vi "Module_p_control_sing_v3.vi"() -> ()   [LabVIEW 2014]
uses:
  <vilib>/rvi/FXPMathLib/FxpSinAndCos/XNode/nifxpmath_SinAndCos.xnode
  <vilib>/eio/EIONode/EIONode.xnode
  <vilib>/rvi/FXPMathLib/FxpMul/XNode/nifxpmath_Multiplier.xnode
  <vilib>/rvi/FXPMathLib/FxpSinAndCos/simVIs/DllFxpSinAndCosTemp_sub.vi
  <vilib>/rvi/FXPMathLib/FxpSinAndCos/subVIs/nifxpmath_SinAndCos_SimConfig.ctl
  <vilib>/rvi/eio/common/nirviEmuTemplateMethod_errors.vi
  <vilib>/rvi/FXPMathLib/sim/FxpSim.dll
  <vilib>/rvi/DataTransferAndStorage/Container/XNode/niFpgaContainer.xnode
  <vilib>/rvi/FXPMathLib/FxpSub/XNode/nifxpmath_Sub.xnode
  <vilib>/rvi/FXPMathLib/FxpAdd/XNode/nifxpmath_Add.xnode
  <vilib>/rvi/Analysis/measure/butterworth/XNode/niFpgaButterworthFilter.xnode
  <vilib>/rvi/FXPMathLib/FxpAtan2/XNode/nifxpmath_Atan2.xnode
  <vilib>/rvi/FXPMathLib/FxpAtan2/simVIs/DllFxpAtan2Temp_sub.vi
  <vilib>/rvi/FXPMathLib/FxpAtan2/subVIs/nifxpmath_Atan2_SimConfig.ctl
  <vilib>/rvi/interface/RandomDataEmulation/nirviRandomDataFpgaMultiElementTemplate.vi
panel:
  in  "fb_limit":fxp<+,16,11>
  in  "Db_d_M_avg_Tc (uSec)":u32 caption="M_avg_Tc (uSec)"
  in  "Method case 2":i32
  out "Omega_b(rad/s)":fxp<+/-,32,18>
  out "Omega_b(M_avg)":fxp<+/-,32,18>
  out "Omega_b(M)":fxp<+/-,32,18>
  in  "Count(s)":u32
  out "Boolean":bool
  out "Db_temp":fxp<+/-,22,7>
  in  "Sin ini":bool
  out "xb_dd":fxp<+/-,25,15>
  in  "scaled coefficients_xb_dd":i32[](array[numeric])=[1067016412, 3362706]
  out "Db_dd":fxp<+/-,25,15>
  in  "scaled coefficients_Db_dd":i32[](array[numeric])=[1067016412, 3362706]
  out "Dab_edd":fxp<+/-,34,12>
  out "Dab_ed":fxp<+/-,33,10>
  out "fbr":fxp<+/-,20,10>
  in  "Kvb":fxp<+,15,8>
  in  "Bvb":fxp<+,15,8>
  out "Dab_e":fxp<+/-,26,11>
  in  "Dbr":fxp<+/-,22,8>
  in  "Inv./Pos.":bool
  out "Dabr_sin/cos":fxp<+/-,22,8>
  in  "Sin_offset_b":fxp<+/-,12,8>
  in  "Sin_magnitude_b":fxp<+/-,11,8>
  out "Dabr_d":fxp<+/-,33,10>
  out "Sin_omega":fxp<+,29,9>
  out "Dabr_dd":fxp<+/-,34,12>
  in  "Sin wave frenqueny (Hz)":fxp<+,21,5>
  out "Db_d(M_avg method)":fxp<+/-,32,12>
  in  "Db_d_M_Tc (mSec)":u32 format="%#_6f"
  out "Db_d(M method)":fxp<+/-,32,12>
  out "xb_d(M_avg method)":fxp<+/-,25,10>
  in  "xb_d_M_avg_Tc (uSec)":u32 caption="M_avg_Tc (uSec)"
  out "xb_d(M method)":fxp<+/-,25,10>
  in  "xb_d_M_Tc (mSec)":u32 format="%#_6f"
  in  "Method case":i32
  out "xb_d(T method)":fxp<+/-,25,10>
  out "Db_d(T method)":fxp<+/-,32,12>
  in  "mt0_velocity":u32
  out "mt_velocity":u32
  in  "mt0_omega":u32
  out "mt_omega":u32
  out "fbt_d":fxp<+/-,25,15>
  out "Db_d(mm/s)":fxp<+/-,32,12>
  out "Atom_Position_b":i32
  out "xb_d(mm/s)":fxp<+/-,25,10>
  in  "dFb_PID_add":bool
  in  "scaled coefficients_dFb_PID":i32[](array[numeric])=[1067016412, 3362706]
  out "dFb_PID":fxp<+/-,25,15>
  out "Sin wave time (s)":fxp<+,64,32>
  in  "Atom Reset_b":bool
  out "xb(mm)":fxp<+/-,22,7>
  in  "Friction tolerance_b":fxp<+,12,4>
  in  "Coe Ini":bool
  in  "Encoder Reset_b":bool
  in  "Stop Motor_b":bool
  in  "viscous_cons_b":fxp<+/-,20,10>
  in  "fstb":fxp<+/-,15,6>
  in  "Db_d_tol":fxp<+,20,12>
  in  "Kib":fxp<+,27,10>
  in  "Kdb":fxp<+,26,2>
  in  "kb c":fxp<+,15,8>
  in  "kb t":fxp<+,15,8>
  out "fbt_i":fxp<+/-,34,18>
  in  "Kpb":fxp<+,11,7>=0.375
  in  "fv_coeff. b":fxp<+,13,1>
  out "Friction comp_b":fxp<+/-,20,10>
  in  "fcb":fxp<+/-,15,6>
  in  "fvb":fxp<+,20,12>
  out "kb":fxp<+,15,8>
  out "fb":fxp<+/-,20,10>
  out "fb_tilde":fxp<+/-,21,11>
  out "Fb_PID":fxp<+/-,21,11>
  in  "fb_tolerance":fxp<+,32,9>=1.0
  out "Encoder Position_b":i32
  out "rad(NrTheta)_b":fxp<+/-,33,18> format="%.21g"
  out "Db(mm)":fxp<+/-,22,7>
  out "Omega_b(T)":fxp<+/-,20,9>
  out "vq_b_F":fxp<+/-,20,5> format="%.57g"
  out "vd_b_F":fxp<+/-,20,5>
  out "va_b":fxp<+/-,20,5> format="%.21g"
  out "vb_b":fxp<+/-,20,5> format="%.21g"
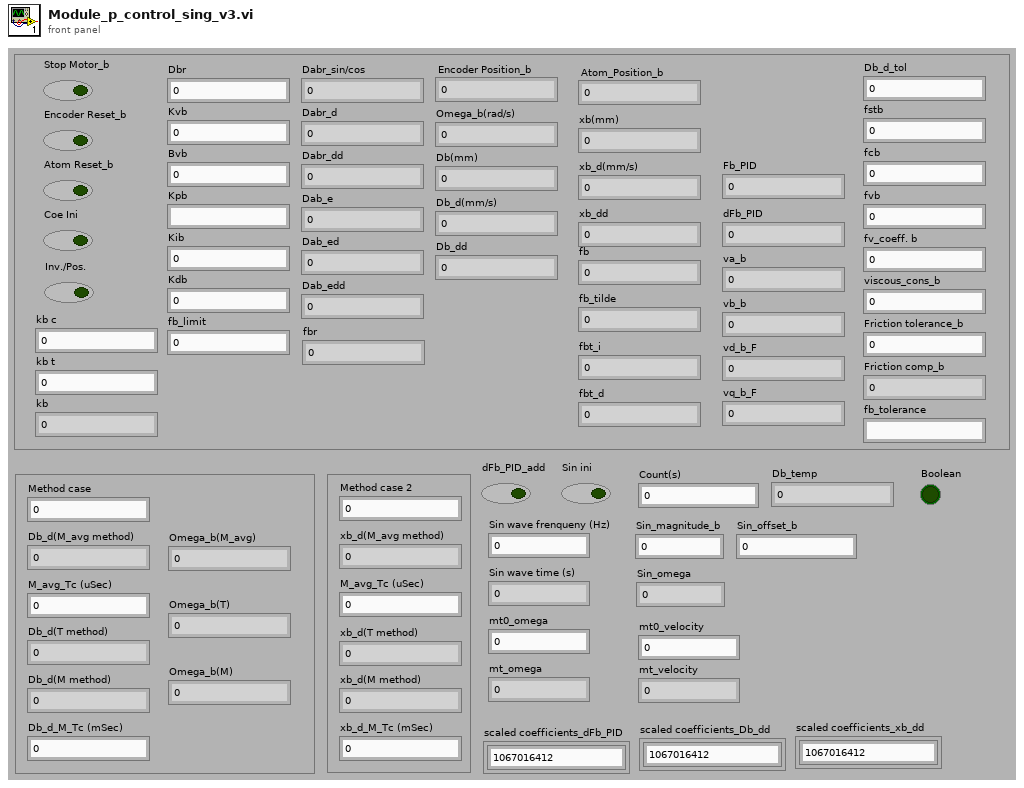
[diagram p1: front panel]
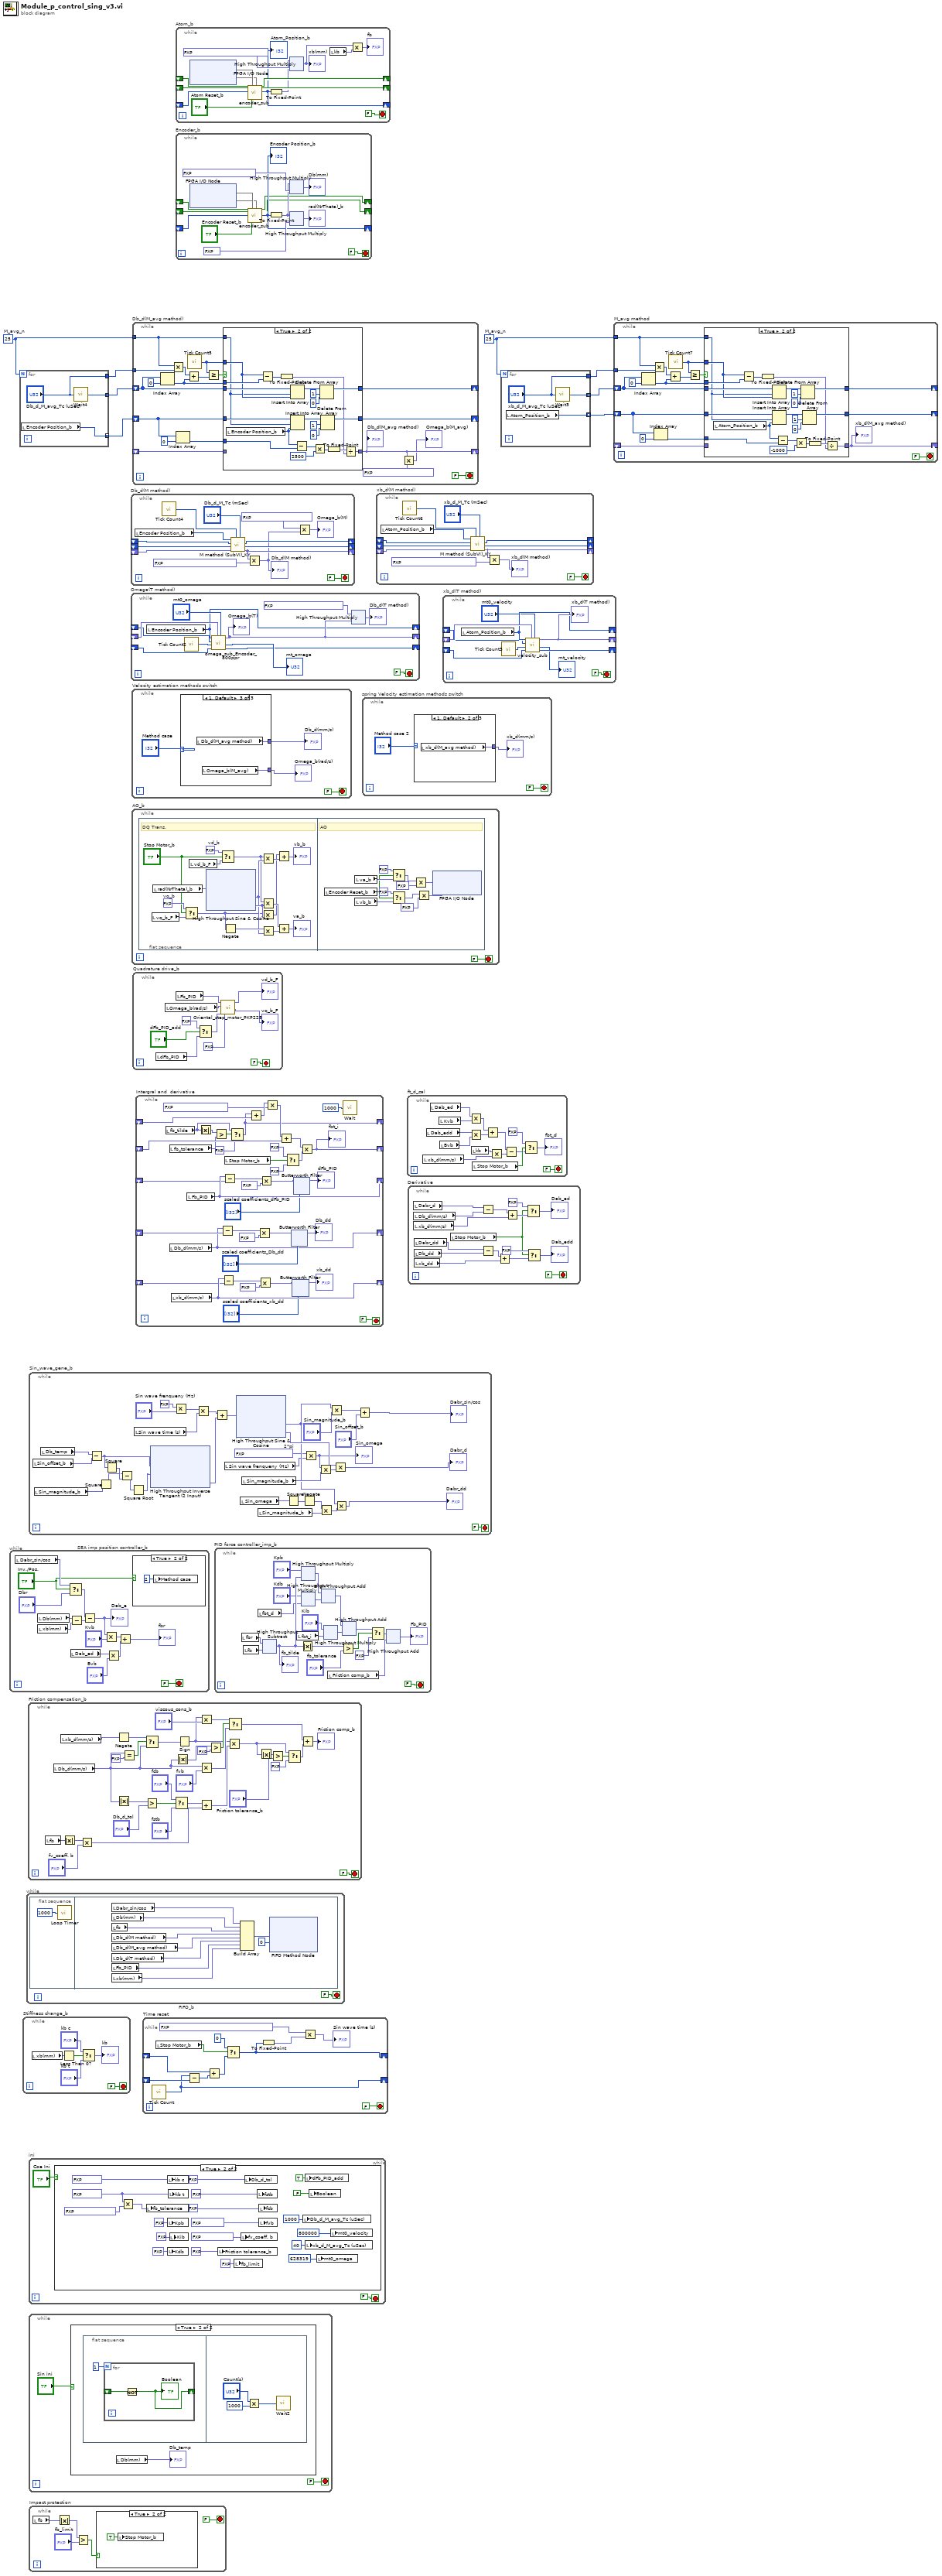
[diagram p0: block diagram]
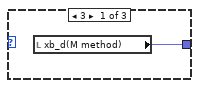
[diagram p4: hidden frame]
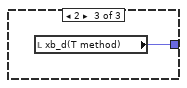
[diagram p5: hidden frame]
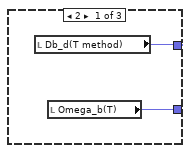
[diagram p9: hidden frame]
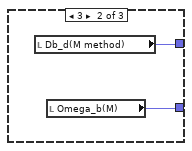
[diagram p10: hidden frame]
diagram:
  w3 = 25  # M_avg_n
  w7 = 25  # M_avg_n
  n1 = while "SEA imp position controller_b" {
    stop <- FALSE stop-if-true
    n2 = local read "Dabr_sin/cos"() -> (w11:fxp<+/-,22,8>)
    n3 = local read "Db(mm)"() -> (w18:fxp<+/-,22,7>)
    n4 = local read "xb(mm)"() -> (w19:fxp<+/-,22,7>)
    n5 = Select(t=w11, s="Inv./Pos.", f="Dbr") -> (s? t:f=w13:fxp<+/-,22,8>)
    n6 = Subtract(x=w18, y=w19) -> (x-y=w17:fxp<+/-,22,7>)
    n7 = local read "Dab_ed"() -> (w16:fxp<+/-,33,10>)
    n8 = Subtract(x=w13, y=w17) -> (x-y=w22:fxp<+/-,24,9>)
    "Dab_e" <- w22
    n9 = Multiply(x=w22, y="Kvb") -> (x*y=w20:fxp<+/-,39,17>)
    n10 = Multiply(x=w16, y="Bvb") -> (x*y=w21:fxp<+/-,48,18>)
    n11 = Add(x=w20, y=w21) -> (x+y=→"fbr":fxp<+/-,20,10>)
    n12 = case shown="True" "Inv./Pos." {
      frame False {
      }
      frame True {
        n13 = local write "Method case"(2 ("Method case")) -> ()
      }
    }
  }
  n14 = for {
    N: w3 -> [_]
    tunnel: [w27] -> w1 mode=indexing
    tunnel: [w25] -> w2 mode=indexing
    tunnel: ["Db_d_M_avg_Tc (uSec)"] -> w4
    n15 = local read "Encoder Position_b"() -> (w25:i32)
    n16 = call "Wait4"("Count(uSec)"="Db_d_M_avg_Tc (uSec)") -> ("Tick Count(uSec)"=w27:u32)
  }
  n17 = while "Stiffness change_b" {
    stop <- FALSE stop-if-true
    n18 = local read "xb(mm)"() -> (w33:fxp<+/-,22,7>)
    n19 = Less Than 0?(x=w33) -> (x < 0?=w32:bool)
    n20 = Select(t="kb c", s=w32, f="kb t") -> (s? t:f=→"kb":fxp<+,15,8>)
  }
  n21 = while "FIFO_b" {
    stop <- FALSE stop-if-true
    n22 = flat-sequence {
      frame #0 {
        n23 = call "Loop Timer"("Count(uSec)"=u32 1000 ("Loop Period (usec)")) -> ()  [unwired: 1 out]
      }
      frame #1 {
        n24 = local read "Dabr_sin/cos"() -> (w41:fxp<+/-,22,8>)
        n25 = local read "Db(mm)"() -> (w40:fxp<+/-,22,7>)
        n26 = local read "fb"() -> (w39:fxp<+/-,20,10>)
        n27 = local read "Db_d(M method)"() -> (w45:fxp<+/-,32,12>)
        n28 = local read "Db_d(M_avg method)"() -> (w38:fxp<+/-,32,12>)
        n29 = local read "Db_d(T method)"() -> (w36:fxp<+/-,32,12>)
        n30 = local read "Fb_PID"() -> (w37:fxp<+/-,21,11>)
        n31 = local read "xb(mm)"() -> (w44:fxp<+/-,22,7>)
        n32 = Build Array(w41, w40, w39, w45, w38, w36, w37, w44) -> (w42:fxp<+/-,32,12>[])
        n33 = xnode ("FIFO Method Node")("Element"=w42, "Timeout"=0) -> ()  [unwired: 1 in, 2 out]
      }
    }
  }
  n34 = while "Friction compensation_b" {
    stop <- FALSE stop-if-true
    n35 = local read "fb"() -> (w75:fxp<+/-,20,10>)
    n36 = local read "Db_d(mm/s)"() -> (w56:fxp<+/-,32,12>)
    n37 = local read "xb_d(mm/s)"() -> (w53:fxp<+/-,25,10>)
    n38 = Absolute Value(x=w75) -> (abs(x)=w76:fxp<+,20,10>)
    n39 = Multiply(x=w76, y="fv_coeff. b") -> (x*y=w73:fxp<+/-,20,10>)
    n40 = Negate(x=w53) -> (-x=w52:fxp<+/-,26,11>)
    n41 = Absolute Value(x=w56) -> (abs(x)=w70:fxp<+,32,12>)
    n42 = Equal?(x=w56, y=fxp<+/-,25,15> 0.0) -> (x = y?=w57:bool)
    n43 = Select(t=w52, s=w57, f=w56) -> (s? t:f=w55:fxp<+/-,32,12>)
    n44 = Greater?(x=w70, y="Db_d_tol") -> (0:w69:bool)
    n45 = Select(t="fcb", s=w69, f="fstb") -> (s? t:f=w67:fxp<+/-,15,6>)
    n46 = Absolute Value(x=w56) -> (abs(x)=w64:fxp<+,32,12>)
    n47 = Sign(1:w55) -> (0:w54:fxp<+/-,2,2>)
    n48 = Multiply(x=w54, y="viscous_cons_b") -> (x*y=w59:fxp<+/-,20,10>)
    n49 = Multiply(x=w56, y="fvb") -> (x*y=w62:fxp<+/-,20,10>)
    n50 = Add(x=w67, y=w73) -> (x+y=w72:fxp<+/-,20,10>)
    n51 = Greater?(x=w64, y=fxp<+/-,25,15> 25.0) -> (0:w63:bool)
    n52 = Multiply(x=w54, y=w72) -> (x*y=w48:fxp<+/-,20,10>)
    n53 = Select(t=w59, s=w63, f=w62) -> (s? t:f=w61:fxp<+/-,20,10>)
    n54 = Absolute Value(x=w48) -> (abs(x)=w50:fxp<+,20,10>)
    n55 = Greater?(x=w50, y="Friction tolerance_b") -> (0:w51:bool)
    n56 = Select(t=w48, s=w51, f=fxp<+/-,20,10> 0.0) -> (s? t:f=w47:fxp<+/-,20,10>)
    n57 = Add(x=w61, y=w47) -> (x+y=→"Friction comp_b":fxp<+/-,20,10>)
  }
  n58 = while "ini" {
    stop <- FALSE stop-if-true
    n59 = case shown="True" "Coe Ini" {
      frame False {
      }
      frame True {
        w92 = fxp<+,15,8> 58.640625 ("kb")
        n60 = Multiply(x=w92, y=fxp<+,17,1> 0.00250244140625 ("kb")) -> (x*y=w93:fxp<+,32,9>)
        n61 = local write "fb_tolerance"(w93) -> ()
        n62 = local write "kb c"(fxp<+,15,8> 58.640625 ("kb")) -> ()
        n63 = local write "Kpb"(fxp<+,11,7> 40.0 ("Kpb")) -> ()
        n64 = local write "Kdb"(fxp<+,26,2> 0.5 ("Kdb")) -> ()
        n65 = local write "kb t"(w92) -> ()
        n66 = local write "Kib"(fxp<+,27,10> 20.0 ("Kib")) -> ()
        n67 = local write "Friction tolerance_b"(fxp<+,12,4> 10.0 ("Friction tolerance_y")) -> ()
        n68 = local write "fb_limit"(fxp<+,10,5> 10.0 ("fb_limit")) -> ()
        n69 = local write "fv_coeff. b"(fxp<+,13,1> 0.14990234375 ("fv_coeff. y")) -> ()
        n70 = local write "Db_d_tol"(fxp<+,20,12> 1.0 ("Dy_d_tol")) -> ()
        n71 = local write "fstb"(fxp<+/-,15,6> 12.0 ("fsty")) -> ()
        n72 = local write "fcb"(fxp<+/-,15,6> 8.0 ("fcy")) -> ()
        n73 = local write "fvb"(fxp<+,20,12> 0.19921875 ("fvy")) -> ()
        n74 = local write "Db_d_M_avg_Tc (uSec)"(u32 1000 ("M_avg_Tc (uSec)")) -> ()
        n75 = local write "dFb_PID_add"(TRUE ("dF_PID_add")) -> ()
        n76 = local write "xb_d_M_avg_Tc (uSec)"(u32 40 ("M_avg_Tc (uSec)")) -> ()
        n77 = local write "Boolean"(FALSE ("dF_PID_add")) -> ()
        n78 = local write "mt0_omega"(u32 628319 ("mt0_omega")) -> ()
        n79 = local write "mt0_velocity"(u32 800000 ("mt0_velocity")) -> ()
      }
    }
  }
  n80 = while {
    stop <- FALSE stop-if-true
    n81 = case shown="True" "Sin ini" {
      frame False {
      }
      frame True {
        n82 = flat-sequence {
          frame #0 {
            n83 = for {
              N: 1 -> [_]
              shift-right: [w106] -> _
              shift-left: _ -> [w107]
              n84 = Not(x=w107) -> (.not. x?=w106:bool)
              "Boolean" <- w106
            }
          }
          frame #1 {
            n85 = Multiply(x="Count(s)", y=u32 1000) -> (x*y=w108:u32)
            n86 = call "Wait2"("Count(mSec)"=w108) -> ()  [unwired: 1 out]
          }
        }
        n87 = local read "Db(mm)"() -> (→"Db_temp":fxp<+/-,22,7>)
      }
    }
  }
  n88 = while "Sin_wave_gene_b" {
    stop <- FALSE stop-if-true
    w116 = fxp<+,20,3> 6.2831878662109375  # 2*pi
    n89 = local read "Sin_offset_b"() -> (w137:fxp<+/-,12,8>)
    n90 = local read "Sin_magnitude_b"() -> (w136:fxp<+/-,11,8>)
    n91 = local read "Db_temp"() -> (w138:fxp<+/-,22,7>)
    n92 = Subtract(x=w138, y=w137) -> (x-y=w135:fxp<+/-,24,9>)
    n93 = Square(x=w136) -> (x^2=w133:fxp<+,21,15>)
    n94 = Square(x=w135) -> (x^2=w134:fxp<+,46,16>)
    n95 = Subtract(x=w133, y=w134) -> (x-y=w132:fxp<+,47,17>)
    n96 = Square Root(x=w132) -> (sqrt(x)=w131:fxp<+,50,9>)
    n97 = local read "Sin wave time (s)"() -> (w118:fxp<+,64,32>)
    n98 = xnode "High Throughput Inverse Tangent (2 Input)"("y"=w135, "x"=w131) -> ("atan2(y,x) (pi)"=w139:fxp<+/-,16,2>)
    n99 = Multiply(x=fxp<+,1,2> 2.0 ("y"), y="Sin wave frenqueny (Hz)") -> (x*y=w119:fxp<+,21,6>)
    n100 = Multiply(x=w119, y=w118) -> (x*y=w117:fxp<+,48,18>)
    n101 = Add(x=w117, y=w139) -> (x+y=w140:fxp<+/-,50,20>)
    n102 = local read "Sin wave frenqueny (Hz)"() -> (w114:fxp<+,21,5>)
    n103 = xnode "High Throughput Sine & Cosine"("x (pi)"=w140) -> ("sin(x)"=w122:fxp<+/-,17,2>, "cos(x)"=w128:fxp<+/-,17,2>)
    n104 = local read "Sin_omega"() -> (w126:fxp<+,29,9>)
    n105 = local read "Sin_magnitude_b"() -> (w130:fxp<+/-,11,8>)
    n106 = local read "Sin_magnitude_b"() -> (w127:fxp<+/-,11,8>)
    n107 = Square(x=w126) -> (x^2=w125:fxp<+,35,15>)
    n108 = Negate(x=w125) -> (-x=w124:fxp<+/-,36,16>)
    n109 = Multiply(x=w116, y=w114) -> (x*y=w115:fxp<+,29,9>)
    "Sin_omega" <- w115
    n110 = Multiply(x=w115, y=w130) -> (x*y=w129:fxp<+,31,9>)
    n111 = Multiply(x=w124, y=w127) -> (x*y=w123:fxp<+/-,34,12>)
    n112 = Multiply(x=w122, y="Sin_magnitude_b") -> (x*y=w143:fxp<+/-,20,8>)
    n113 = Multiply(x=w128, y=w129) -> (x*y=→"Dabr_d":fxp<+/-,33,10>)
    n114 = Multiply(x=w122, y=w123) -> (x*y=→"Dabr_dd":fxp<+/-,34,12>)
    n115 = Add(x=w143, y="Sin_offset_b") -> (x+y=→"Dabr_sin/cos":fxp<+/-,22,8>)
  }
  n116 = while "Impact protection" {
    stop <- FALSE stop-if-true
    n117 = local read "fb"() -> (w206:fxp<+/-,20,10>)
    n118 = Absolute Value(x=w206) -> (abs(x)=w205:fxp<+,20,10>)
    n119 = Greater?(x=w205, y="fb_limit") -> (0:w203:bool)
    n120 = case shown="True" w203 {
      frame False {
      }
      frame True {
        n121 = local write "Stop Motor_b"(TRUE ("Stop Motor_b")) -> ()
      }
    }
  }
  n122 = while "Db_d(M method)" {
    shift-right: [w220] -> _
    shift-left: _ -> [w215]
    shift-right: [w219] -> _
    shift-left: _ -> [w214]
    shift-right: [w212] -> _
    shift-left: _ -> [w213]
    stop <- FALSE stop-if-true
    n123 = local read "Encoder Position_b"() -> (w216:i32)
    n124 = call "Tick Count4"() -> ("Tick Count(mSec)"=w217:u32)
    n125 = call "M method (SubVI)_KY.vi"("Tc (mSec)"="Db_d_M_Tc (mSec)", "Tick Count (mSec)"=w217, "Encoder velocity_pre (pulse/s)"=w213, "Shift Register in 2"=w214, "Shift Register in 1"=w215, "Encoder pulses"=w216) -> ("Encoder velocity (pulse/s)"=w212:fxp<+/-,64,32>, "Shift Register out 2"=w219:i32, "Shift Register out 1"=w220:u32)  [unwired: 3 in]
    n126 = Multiply(x=w212, y=fxp<+/-,20,-5> 0.002499997615814209) -> (x*y=w211:fxp<+/-,32,12>)
    "Db_d(M method)" <- w211
    n127 = Multiply(x=fxp<+/-,32,12> 3.1415929794311523, y=w211) -> (x*y=→"Omega_b(M)":fxp<+/-,32,18>)
  }
  n128 = while "Omega(T method)" {
    shift-right: [w225] -> _
    shift-left: _ -> [w224]
    shift-right: [w223] -> _
    shift-left: _ -> [w230]
    shift-right: [w228] -> _
    shift-left: _ -> [w226]
    stop <- FALSE stop-if-true
    n129 = local read "Encoder Position_b"() -> (w225:i32)
    n130 = call "Tick Count2"() -> ("Tick Count(Ticks)"=w231:u32)
    n131 = call "omega_sub_Encoder_800ppr.vi"("mt0"="mt0_omega", "omega_pre"=w226, "ticks_m_pre"=w230, "ticks"=w231, "count_pre"=w224, "count"=w225) -> ("ticks_m"=w223:u32, "mt"=→"mt_omega":u32, "omega"=w228:fxp<+/-,20,9>)  [unwired: 3 in]
    "Omega_b(T)" <- w228
    n132 = xnode ("High Throughput Multiply")("x"=fxp<+/-,26,1> 0.3183099031448364, "y"=w228) -> ("x*y"=→"Db_d(T method)":fxp<+/-,32,12>)
  }
  n133 = while "Velocity estimation methods switch" {
    stop <- FALSE stop-if-true
    n134 = case shown="1, Default" "Method case" {
      tunnel: [w239 w241 w243] -> w236
      tunnel: [w240 w242 w244] -> w235
      frame 2 {
        n135 = local read "Db_d(T method)"() -> (w239:fxp<+/-,32,12>)
        n136 = local read "Omega_b(T)"() -> (w240:fxp<+/-,20,9>)
      }
      frame 3 {
        n137 = local read "Db_d(M method)"() -> (w241:fxp<+/-,32,12>)
        n138 = local read "Omega_b(M)"() -> (w242:fxp<+/-,32,18>)
      }
      frame 1, Default {
        n139 = local read "Db_d(M_avg method)"() -> (w243:fxp<+/-,32,12>)
        n140 = local read "Omega_b(M_avg)"() -> (w244:fxp<+/-,32,18>)
      }
    }
    "Db_d(mm/s)" <- w236
    "Omega_b(rad/s)" <- w235
  }
  n141 = while "AO_b" {
    stop <- FALSE stop-if-true
    n142 = flat-sequence {
      frame #0 {
        w252 = fxp<+/-,20,5> 0.0  # vq_b
        w251 = fxp<+/-,20,5> 0.0  # vd_b
        # "DQ Trans."
        n143 = local read "vq_b_F"() -> (w249:fxp<+/-,20,5>)
        n144 = local read "rad(NrTheta)_b"() -> (w262:fxp<+/-,33,18>)
        n145 = Select(t=w252, s="Stop Motor_b", f=w249) -> (s? t:f=w246:fxp<+/-,20,5>)
        n146 = local read "vd_b_F"() -> (w250:fxp<+/-,20,5>)
        n147 = xnode "High Throughput Sine & Cosine"("x (pi)"=w262) -> ("sin(x)"=w253:fxp<+/-,17,2>, "cos(x)"=w254:fxp<+/-,17,2>)
        n148 = Select(t=w251, s="Stop Motor_b", f=w250) -> (s? t:f=w247:fxp<+/-,20,5>)
        n149 = Negate(x=w246) -> (-x=w261:fxp<+/-,21,6>)
        n150 = Multiply(x=w247, y=w253) -> (x*y=w257:fxp<+/-,20,5>)
        n151 = Multiply(x=w247, y=w254) -> (x*y=w260:fxp<+/-,20,5>)
        n152 = Multiply(x=w246, y=w254) -> (x*y=w256:fxp<+/-,20,5>)
        n153 = Multiply(x=w261, y=w253) -> (x*y=w259:fxp<+/-,20,5>)
        n154 = Add(x=w256, y=w257) -> (x+y=→"vb_b":fxp<+/-,20,5>)
        n155 = Add(x=w260, y=w259) -> (x+y=→"va_b":fxp<+/-,20,5>)
      }
      frame #1 {
        # "AO"
        n156 = local read "Encoder Reset_b"() -> (w299:bool)
        n157 = local read "va_b"() -> (w300:fxp<+/-,20,5>)
        n158 = local read "vb_b"() -> (w301:fxp<+/-,20,5>)
        n159 = Select(t=fxp<+/-,20,5> 3.0 ("Mod2/AO4"), s=w299, f=w300) -> (s? t:f=w297:fxp<+/-,20,5>)
        n160 = Select(t=fxp<+/-,20,5> 0.0 ("Mod2/AO4"), s=w299, f=w301) -> (s? t:f=w294:fxp<+/-,20,5>)
        n161 = Multiply(x=w297, y=fxp<+/-,20,5> -0.5) -> (x*y=w298:fxp<+/-,20,5>)
        n162 = Multiply(x=w294, y=fxp<+/-,20,5> -0.5) -> (x*y=w293:fxp<+/-,20,5>)
        n163 = xnode "FPGA I/O Node"("Mod2/AO0"=w298, "Mod2/AO1"=w293) -> ()  [unwired: 2 in, 2 out]
      }
    }
  }
  n164 = while "Db_d(M_avg method)" {
    shift-right: [w314] -> _
    shift-left: w1 -> [w317]
    tunnel: w3 -> [w315]
    shift-right: [w312] -> _
    shift-left: w2 -> [w310]
    shift-right: [w305] -> _
    shift-left: _ -> [w308]
    tunnel: w4 -> [w307]
    stop <- FALSE stop-if-true
    n165 = Index Array(array=w317, index=0) -> (element=w313:u32)
    n166 = Multiply(x=w315, y=w307) -> (x*y=w320:u32)
    n167 = Index Array(array=w310, index=0) -> (element=w309:i32)
    n168 = Add(x=w320, y=w313) -> (x+y=w319:u32)
    n169 = call "Tick Count5"() -> ("Tick Count(uSec)"=w316:u32)
    n170 = Greater Or Equal?(x=w316, y=w319) -> (x >= y?=w318:bool)
    n171 = case shown="True" w318 {
      tunnel: w317 -> [w325 w347]
      tunnel: w316 -> [_ w341]
      tunnel: w315 -> [_ w330]
      tunnel: [w325 w343] -> w314
      tunnel: w313 -> [_ w342]
      tunnel: w310 -> [w324 w331]
      tunnel: [w324 w329] -> w312
      tunnel: [w323 w328] -> w305
      tunnel: w309 -> [_ w326]
      tunnel: w308 -> [w323 _]
      frame False {
      }
      frame True {
        n172 = local read "Encoder Position_b"() -> (w335:i32)
        n173 = Subtract(x=w341, y=w342) -> (x-y=w340:u32)
        n174 = To Fixed-Point(number=w340) -> (fixed-point=w327:fxp<+,32,32>)  [unwired: 1 in]
        n175 = Insert Into Array(array=w347, index=w330, new element=w341) -> (w346:u32[])
        n176 = Insert Into Array(array=w331, index=w330, new element=w335) -> (w332:i32[])
        n177 = Subtract(x=w335, y=w326) -> (x-y=w336:i32)
        n178 = Multiply(x=w336, y=2500) -> (x*y=w338:i32)
        n179 = Delete From Array(array=w346, length=1, index=0) -> (array with subset deleted=w343:u32[])  [unwired: 1 out]
        n180 = Delete From Array(array=w332, length=1, index=0) -> (array with subset deleted=w329:i32[])  [unwired: 1 out]
        n181 = To Fixed-Point(number=w338) -> (fixed-point=w339:fxp<+/-,32,32>)  [unwired: 1 in]
        n182 = Divide(x=w339, y=w327) -> (x/y=w328:fxp<+/-,32,12>)
      }
    }
    "Db_d(M_avg method)" <- w305
    n183 = Multiply(x=w305, y=fxp<+/-,32,12> 3.1415929794311523 ("x")) -> (x*y=→"Omega_b(M_avg)":fxp<+/-,32,18>)
  }
  n184 = while "Quadrature drive_b" {
    stop <- FALSE stop-if-true
    n185 = local read "dFb_PID"() -> (w354:fxp<+/-,25,15>)
    n186 = local read "Omega_b(rad/s)"() -> (w350:fxp<+/-,32,18>)
    n187 = local read "Fb_PID"() -> (w351:fxp<+/-,21,11>)
    n188 = Select(t=fxp<+/-,25,15> 0.0 ("f"), s="dFb_PID_add", f=w354) -> (s? t:f=w349:fxp<+/-,25,15>)
    n189 = call "Oriental_step_motor_PKP225.vi"("F_Threshold"=fxp<+,12,12> 10.0, "dFmr"=w349, "omega"=w350, "Fmr"=w351) -> ("vq_F"=→"vq_b_F":fxp<+/-,20,5>, "vd_F"=→"vd_b_F":fxp<+/-,20,5>)  [unwired: 6 in]
  }
  n190 = while "Intergral and  derivative" {
    shift-right: [w385] -> _
    shift-left: _ -> [w386]
    shift-right: [w372] -> _
    shift-left: _ -> [w391]
    shift-right: [w381] -> _
    shift-left: _ -> [w379]
    shift-right: [w365] -> _
    shift-left: _ -> [w366]
    shift-right: [w364] -> _
    shift-left: _ -> [w363]
    stop <- FALSE stop-if-true
    n191 = local read "fb_tilde"() -> (w387:fxp<+/-,21,11>)
    n192 = local read "fb_tolerance"() -> (w389:fxp<+,32,9>)
    n193 = local read "Db_d(mm/s)"() -> (w365:fxp<+/-,32,12>)
    n194 = local read "xb_d(mm/s)"() -> (w364:fxp<+/-,25,10>)
    n195 = local read "Fb_PID"() -> (w381:fxp<+/-,21,11>)
    n196 = Absolute Value(x=w387) -> (abs(x)=w390:fxp<+,21,11>)
    n197 = Greater?(x=w390, y=w389) -> (0:w388:bool)
    n198 = Subtract(x=w365, y=w366) -> (x-y=w368:fxp<+/-,33,13>)
    n199 = Subtract(x=w364, y=w363) -> (x-y=w361:fxp<+/-,26,11>)
    n200 = Subtract(x=w381, y=w379) -> (x-y=w380:fxp<+/-,22,12>)
    n201 = local read "Stop Motor_b"() -> (w393:bool)
    n202 = Select(t=w387, s=w388, f=fxp<+/-,21,11> 0.0) -> (s? t:f=w385:fxp<+/-,21,11>)
    n203 = Add(x=w385, y=w386) -> (x+y=w395:fxp<+/-,22,12>)
    n204 = Multiply(x=w368, y=fxp<+,10,10> 1000.0) -> (x*y=w369:fxp<+/-,25,15>)
    n205 = Multiply(x=w361, y=fxp<+,10,10> 1000.0) -> (x*y=w360:fxp<+/-,25,15>)
    n206 = Multiply(x=w380, y=fxp<+,10,10> 1000.0) -> (x*y=w378:fxp<+/-,25,15>)
    n207 = Multiply(x=w395, y=fxp<+/-,30,12> 0.000499725341796875) -> (x*y=w392:fxp<+/-,25,15>)
    n208 = Add(x=w392, y=w391) -> (x+y=w373:fxp<+/-,32,16>)
    n209 = Select(t=fxp<+/-,2,2> 0.0, s=w393, f=fxp<+/-,2,2> 1.0) -> (s? t:f=w374:fxp<+/-,2,2>)
    n210 = xnode "Butterworth Filter"("input data"=w369, "scaled coefficients"="scaled coefficients_Db_dd") -> ("output data"=→"Db_dd":fxp<+/-,25,15>)  [unwired: 1 in]
    n211 = xnode "Butterworth Filter"("input data"=w360, "scaled coefficients"="scaled coefficients_xb_dd") -> ("output data"=→"xb_dd":fxp<+/-,25,15>)  [unwired: 1 in]
    n212 = xnode "Butterworth Filter"("input data"=w378, "scaled coefficients"="scaled coefficients_dFb_PID") -> ("output data"=→"dFb_PID":fxp<+/-,25,15>)  [unwired: 1 in]
    n213 = Multiply(x=w373, y=w374) -> (x*y=w372:fxp<+/-,34,18>)
    "fbt_i" <- w372
    n214 = call "Wait"("Count(uSec)"=u32 1000 ("Count(mSec)")) -> ()  [unwired: 1 out]
  }
  n215 = while "Time reset" {
    shift-right: [w432] -> _
    shift-left: _ -> [w433]
    shift-right: [w424] -> _
    shift-left: _ -> [w426]
    stop <- FALSE stop-if-true
    n216 = call "Tick Count"() -> ("Tick Count(uSec)"=w432:u32)
    n217 = local read "Stop Motor_b"() -> (w429:bool)
    n218 = Subtract(x=w432, y=w433) -> (x-y=w428:u32)
    n219 = Add(x=w426, y=w428) -> (x+y=w427:u32)
    n220 = Select(t=u32 0, s=w429, f=w427) -> (s? t:f=w424:u32)
    n221 = To Fixed-Point(number=w424) -> (fixed-point=w422:fxp<+,64,32>)  [unwired: 1 in]
    n222 = Multiply(x=fxp<+,20,-18> 1.0000003385357559e-06 ("y"), y=w422) -> (x*y=→"Sin wave time (s)":fxp<+,64,32>)
  }
  n223 = while "Atom_b" {
    shift-right: [w447] -> _
    shift-left: _ -> [w445]
    shift-right: [w446] -> _
    shift-left: _ -> [w444]
    shift-right: [w434] -> _
    shift-left: _ -> [w441]
    stop <- FALSE stop-if-true
    n224 = xnode "FPGA I/O Node"() -> ("Mod5/DI0"=w443, "Mod5/DI1"=w442)  [unwired: 2 in, 2 out]
    n225 = call "encoder_sub.vi"("A_pre"=w445, "B_pre"=w444, "Encoder Position_pre"=w441, "A input"=w443, "Encoder Position Reset"="Atom Reset_b", "B input"=w442) -> ("A"=w447:bool, "B"=w446:bool, "Encoder Position (Counts)"=w434:i32)  [unwired: 19 in]
    "Atom_Position_b" <- w434
    n226 = To Fixed-Point(number=w434) -> (fixed-point=w439:fxp<+/-,18,18>)  [unwired: 1 in]
    n227 = xnode ("High Throughput Multiply")("x"=w439, "y"=fxp<+/-,20,-5> -0.0009999871253967285) -> ("x*y"=w436:fxp<+/-,22,7>)
    "xb(mm)" <- w436
    n228 = local read "kb"() -> (w437:fxp<+,15,8>)
    n229 = Multiply(x=w436, y=w437) -> (x*y=→"fb":fxp<+/-,20,10>)
  }
  n230 = while "Encoder_b" {
    shift-right: [w450] -> _
    shift-left: _ -> [w462]
    shift-right: [w449] -> _
    shift-left: _ -> [w461]
    shift-right: [w454] -> _
    shift-left: _ -> [w460]
    stop <- FALSE stop-if-true
    n231 = xnode "FPGA I/O Node"() -> ("Mod5/DI3"=w452, "Mod5/DI4"=w451)  [unwired: 2 in, 2 out]
    n232 = call "encoder_sub.vi"("A_pre"=w462, "B_pre"=w461, "Encoder Position_pre"=w460, "A input"=w452, "Encoder Position Reset"="Encoder Reset_b", "B input"=w451) -> ("A"=w450:bool, "B"=w449:bool, "Encoder Position (Counts)"=w454:i32)  [unwired: 19 in]
    "Encoder Position_b" <- w454
    n233 = To Fixed-Point(number=w454) -> (fixed-point=w457:fxp<+/-,18,18>)  [unwired: 1 in]
    n234 = xnode ("High Throughput Multiply")("x"=w457, "y"=fxp<+/-,15,-7> 0.0025000572204589844) -> ("x*y"=→"Db(mm)":fxp<+/-,22,7>)
    n235 = xnode ("High Throughput Multiply")("x"=w457, "y"=fxp<+,24,0> 0.125) -> ("x*y"=→"rad(NrTheta)_b":fxp<+/-,33,18>)
  }
  n236 = while "PID force controller_imp_b" {
    stop <- FALSE stop-if-true
    n237 = local read "fbr"() -> (w467:fxp<+/-,20,10>)
    n238 = local read "fb"() -> (w478:fxp<+/-,20,10>)
    n239 = local read "fbt_d"() -> (w465:fxp<+/-,25,15>)
    n240 = xnode "High Throughput Subtract"("x"=w467, "y"=w478) -> ("x-y"=w480:fxp<+/-,21,11>)
    "fb_tilde" <- w480
    n241 = local read "fbt_i"() -> (w476:fxp<+/-,34,18>)
    n242 = Absolute Value(x=w480) -> (abs(x)=w482:fxp<+,21,11>)
    n243 = xnode ("High Throughput Multiply")("x"="Kpb", "y"=w480) -> ("x*y"=w479:fxp<+/-,33,17>)
    n244 = xnode ("High Throughput Multiply")("x"="Kdb", "y"=w465) -> ("x*y"=w473:fxp<+/-,31,21>)
    n245 = xnode ("High Throughput Add")("x"=w479, "y"=w473) -> ("x+y"=w477:fxp<+/-,21,11>)
    n246 = xnode ("High Throughput Multiply")("x"="Kib", "y"=w476) -> ("x*y"=w475:fxp<+/-,31,14>)
    n247 = local read "Friction comp_b"() -> (w471:fxp<+/-,20,10>)
    n248 = Greater?(x=w482, y="fb_tolerance") -> (0:w481:bool)
    n249 = xnode ("High Throughput Add")("x"=w477, "y"=w475) -> ("x+y"=w474:fxp<+/-,21,11>)
    n250 = Select(t=w474, s=w481, f=fxp<+/-,21,11> 0.0) -> (s? t:f=w472:fxp<+/-,21,11>)
    n251 = xnode ("High Throughput Add")("x"=w472, "y"=w471) -> ("x+y"=→"Fb_PID":fxp<+/-,21,11>)
  }
  n252 = while "spring Velocity estimation methods switch" {
    stop <- FALSE stop-if-true
    n253 = case shown="1, Default" "Method case 2" {
      tunnel: [w488 w489 w490] -> w485
      frame 3 {
        n254 = local read "xb_d(M method)"() -> (w488:fxp<+/-,25,10>)
      }
      frame 1, Default {
        n255 = local read "xb_d(M_avg method)"() -> (w489:fxp<+/-,25,10>)
      }
      frame 2 {
        n256 = local read "xb_d(T method)"() -> (w490:fxp<+/-,25,10>)
      }
    }
    "xb_d(mm/s)" <- w485
  }
  n257 = while "xb_d(M method)" {
    shift-right: [w499] -> _
    shift-left: _ -> [w494]
    shift-right: [w498] -> _
    shift-left: _ -> [w493]
    shift-right: [w491] -> _
    shift-left: _ -> [w492]
    stop <- FALSE stop-if-true
    n258 = local read "Atom_Position_b"() -> (w495:i32)
    n259 = call "Tick Count6"() -> ("Tick Count(mSec)"=w496:u32)
    n260 = call "M method (SubVI)_KY.vi"("Tc (mSec)"="xb_d_M_Tc (mSec)", "Tick Count (mSec)"=w496, "Encoder velocity_pre (pulse/s)"=w492, "Shift Register in 2"=w493, "Shift Register in 1"=w494, "Encoder pulses"=w495) -> ("Encoder velocity (pulse/s)"=w491:fxp<+/-,64,32>, "Shift Register out 2"=w498:i32, "Shift Register out 1"=w499:u32)  [unwired: 3 in]
    n261 = Multiply(x=w491, y=fxp<+/-,20,-5> -0.0009999871253967285) -> (x*y=→"xb_d(M method)":fxp<+/-,25,10>)
  }
  n262 = while "ft_d_cal" {
    stop <- FALSE stop-if-true
    n263 = local read "xb_d(mm/s)"() -> (w515:fxp<+/-,25,10>)
    n264 = local read "Dab_edd"() -> (w509:fxp<+/-,34,12>)
    n265 = local read "Dab_ed"() -> (w510:fxp<+/-,33,10>)
    n266 = local read "Kvb"() -> (w508:fxp<+,15,8>)
    n267 = local read "Bvb"() -> (w507:fxp<+,15,8>)
    n268 = Multiply(x=w510, y=w508) -> (x*y=w512:fxp<+/-,48,18>)
    n269 = Multiply(x=w509, y=w507) -> (x*y=w513:fxp<+/-,49,20>)
    n270 = local read "kb"() -> (w516:fxp<+,15,8>)
    n271 = local read "Stop Motor_b"() -> (w506:bool)
    n272 = Add(x=w512, y=w513) -> (x+y=w514:fxp<+/-,51,21>)
    n273 = Multiply(x=w516, y=w515) -> (x*y=w517:fxp<+/-,35,12>)
    n274 = Subtract(x=w514, y=w517) -> (x-y=w505:fxp<+/-,25,15>)
    n275 = Select(t=fxp<+/-,25,15> 0.0, s=w506, f=w505) -> (s? t:f=→"fbt_d":fxp<+/-,25,15>)
  }
  n276 = while "Derivative" {
    stop <- FALSE stop-if-true
    n277 = local read "Dabr_d"() -> (w530:fxp<+/-,33,10>)
    n278 = local read "Db_d(mm/s)"() -> (w531:fxp<+/-,32,12>)
    n279 = local read "xb_d(mm/s)"() -> (w533:fxp<+/-,25,10>)
    n280 = local read "Dabr_dd"() -> (w528:fxp<+/-,34,12>)
    n281 = local read "Db_dd"() -> (w527:fxp<+/-,25,15>)
    n282 = local read "xb_dd"() -> (w525:fxp<+/-,25,15>)
    n283 = local read "Stop Motor_b"() -> (w518:bool)
    n284 = Subtract(x=w530, y=w531) -> (x-y=w532:fxp<+/-,33,10>)
    n285 = Subtract(x=w528, y=w527) -> (x-y=w526:fxp<+/-,38,16>)
    n286 = Add(x=w526, y=w525) -> (x+y=w522:fxp<+/-,34,12>)
    n287 = Add(x=w532, y=w533) -> (x+y=w524:fxp<+/-,33,10>)
    n288 = Select(t=fxp<+/-,33,10> 0.0, s=w518, f=w524) -> (s? t:f=→"Dab_ed":fxp<+/-,33,10>)
    n289 = Select(t=fxp<+/-,34,12> 0.0, s=w518, f=w522) -> (s? t:f=→"Dab_edd":fxp<+/-,34,12>)
  }
  n290 = while "xb_d(T method)" {
    shift-right: [w539] -> _
    shift-left: _ -> [w538]
    shift-right: [w541] -> _
    shift-left: _ -> [w536]
    shift-right: [w542] -> _
    shift-left: _ -> [w540]
    stop <- FALSE stop-if-true
    n291 = local read "Atom_Position_b"() -> (w539:i32)
    n292 = call "Tick Count3"() -> ("Tick Count(Ticks)"=w537:u32)
    n293 = call "velocity_sub.vi"("mt0"="mt0_velocity", "velocity_pre"=w540, "ticks_m_pre"=w536, "ticks"=w537, "count_pre"=w538, "count"=w539) -> ("ticks_m"=w541:u32, "mt"=→"mt_velocity":u32, "velocity (mm/s)"=w542:fxp<+/-,25,10>)  [unwired: 3 in]
    "xb_d(T method)" <- w542
  }
  n294 = for {
    N: w7 -> [_]
    tunnel: [w546] -> w8 mode=indexing
    tunnel: ["xb_d_M_avg_Tc (uSec)"] -> w6
    tunnel: [w544] -> w5 mode=indexing
    n295 = local read "Atom_Position_b"() -> (w544:i32)
    n296 = call "Wait3"("Count(uSec)"="xb_d_M_avg_Tc (uSec)") -> ("Tick Count(uSec)"=w546:u32)
  }
  n297 = while "M_avg method" {
    shift-right: [w554] -> _
    shift-left: w8 -> [w557]
    shift-right: [w548] -> _
    shift-left: w5 -> [w551]
    tunnel: w7 -> [w555]
    shift-right: [w550] -> _
    shift-left: _ -> [w549]
    tunnel: w6 -> [w547]
    stop <- FALSE stop-if-true
    n298 = Index Array(array=w557, index=0) -> (element=w553:u32)
    n299 = Multiply(x=w555, y=w547) -> (x*y=w560:u32)
    n300 = Index Array(array=w551, index=0) -> (element=w552:i32)
    n301 = Add(x=w560, y=w553) -> (x+y=w559:u32)
    n302 = call "Tick Count7"() -> ("Tick Count(uSec)"=w556:u32)
    n303 = Greater Or Equal?(x=w556, y=w559) -> (x >= y?=w558:bool)
    n304 = case shown="True" w558 {
      tunnel: w557 -> [w566 w588]
      tunnel: w556 -> [_ w582]
      tunnel: w555 -> [_ w568]
      tunnel: [w566 w584] -> w554
      tunnel: w553 -> [_ w583]
      tunnel: w551 -> [w565 w579]
      tunnel: w552 -> [_ w575]
      tunnel: [w564 w570] -> w550
      tunnel: w549 -> [w564 _]
      tunnel: [w565 w569] -> w548
      frame False {
      }
      frame True {
        n305 = local read "Atom_Position_b"() -> (w576:i32)
        n306 = Subtract(x=w582, y=w583) -> (x-y=w581:u32)
        n307 = To Fixed-Point(number=w581) -> (fixed-point=w567:fxp<+,32,32>)  [unwired: 1 in]
        n308 = Insert Into Array(array=w588, index=w568, new element=w582) -> (w587:u32[])
        n309 = Insert Into Array(array=w579, index=w568, new element=w576) -> (w580:i32[])
        n310 = Subtract(x=w576, y=w575) -> (x-y=w574:i32)
        n311 = Multiply(x=w574, y=-1000) -> (x*y=w572:i32)
        n312 = Delete From Array(array=w587, length=1, index=0) -> (array with subset deleted=w584:u32[])  [unwired: 1 out]
        n313 = Delete From Array(array=w580, length=1, index=0) -> (array with subset deleted=w569:i32[])  [unwired: 1 out]
        n314 = To Fixed-Point(number=w572) -> (fixed-point=w571:fxp<+/-,32,32>)  [unwired: 1 in]
        n315 = Divide(x=w571, y=w567) -> (x/y=w570:fxp<+/-,25,10>)
      }
    }
    "xb_d(M_avg method)" <- w550
  }
